vi "UNIXTime.vi"(8 "error in (no error)":errorcluster) -> (0 "error out":errorcluster, 2 "IntUnixTime 4":i32, 3 "Unix time 4":dbl format="%#_13g")   [LabVIEW 2015]
uses:
  kernel32.dll
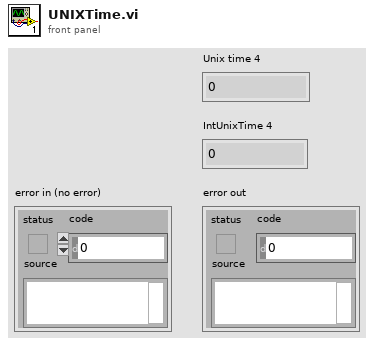
[diagram p1: front panel]
types:
  T1 = cluster{"[0]":u16, "[1]":u16, "[2]":u16, "[3]":u16, "[4]":u16, "[5]":u16, "[6]":u16, "[7]":u16, "[8]":u16, "[9]":u16, "[10]":u16, "[11]":u16, "[12]":u16, "[13]":u16, "[14]":u16, "[15]":u16, "[16]":u16, "[17]":u16, "[18]":u16, "[19]":u16, "[20]":u16, "[21]":u16, "[22]":u16, "[23]":u16, "[24]":u16, "[25]":u16, "[26]":u16, "[27]":u16, "[28]":u16, "[29]":u16, "[30]":u16, "[31]":u16, "[32]":u16, "[33]":u16, "[34]":u16, "[35]":u16, "[36]":u16, "[37]":u16, "[38]":u16, "[39]":u16, "[40]":u16, "[41]":u16, "[42]":u16, "[43]":u16, "[44]":u16, "[45]":u16, "[46]":u16, "[47]":u16, "[48]":u16, "[49]":u16, "[50]":u16, "[51]":u16, "[52]":u16, "[53]":u16, "[54]":u16, "[55]":u16, "[56]":u16, "[57]":u16, "[58]":u16, "[59]":u16, "[60]":u16, "[61]":u16, "[62]":u16, "[63]":u16, "[64]":u16, "[65]":u16, "[66]":u16, "[67]":u16, "[68]":u16, "[69]":u16, "[70]":u16, "[71]":u16, "[72]":u16, "[73]":u16, "[74]":u16, "[75]":u16, "[76]":u16, "[77]":u16, "[78]":u16, "[79]":u16, "[80]":u16, "[81]":u16, "[82]":u16, "[83]":u16, "[84]":u16, "[85]":u16}
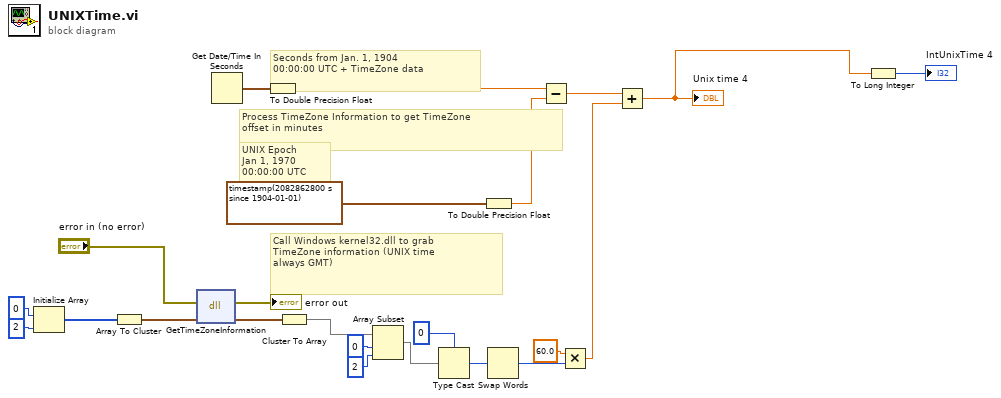
[diagram p0: block diagram]
diagram:
  # "Seconds from Jan. 1, 1904\n00:00:00 UTC + TimeZone data"
  # "UNIX Epoch\nJan 1, 1970\n00:00:00 UTC"
  # "Process TimeZone Information to get TimeZone\noffset in minutes"
  # "Call Windows kernel32.dll to grab\nTimeZone information (UNIX time\nalways GMT)"
  n1 = Initialize Array(u16 0 ("element"), 2 ("dimension size")) -> (w5:u16[])
  n2 = Array To Cluster(array=w5) -> (cluster=w8:T1)
  n3 = dll-call lib="kernel32.dll" fn="GetTimeZoneInformation"(error in="error in (no error)", "lpTimeZoneInformation"=w8) -> (error out=→"error out":errorcluster, "lpTimeZoneInformation"=w9:T1)  [unwired: 2 in, 2 out]
  n4 = Get Date/Time In Seconds() -> (seconds since 1Jan1904=w1:timestamp)
  n5 = To Double Precision Float(number=w1) -> (double precision float=w3:dbl)
  n6 = Cluster To Array(cluster=w9) -> (array=w10:u16[])
  n7 = Array Subset(array=w10, index=0, length=2) -> (w14:u16[])
  n8 = Type Cast(type=0, x=w14) -> (*(type *) &x=w15:i32)
  n9 = To Double Precision Float(number=timestamp(2082862800 s since 1904-01-01)) -> (double precision float=w4:dbl)
  n10 = Swap Words(1:w15) -> (0:w18:i32)
  n11 = Subtract(x=w3, y=w4) -> (x-y=w16:dbl)
  n12 = Multiply(x=60.0 ("y"), y=w18) -> (x*y=w17:dbl)
  n13 = Add(x=w16, y=w17) -> (x+y=w22:dbl)
  "Unix time 4" <- w22
  n14 = To Long Integer(number=w22) -> (32bit integer=→"IntUnixTime 4":i32)
